vi "Restore Cursor Property.vi"(4 "Control Ref Cluster":T1, 6 "Update?":bool=TRUE, 8 "error in (no error)":errorcluster, 11 "2D Plot.lvclass in":refnum<class "2D Plot.lvclass">) -> (0 "error out":errorcluster, 3 "2D Plot.lvclass out":refnum<class "2D Plot.lvclass">)   [LabVIEW 2017, in "2D Plot.lvclass"]
uses:
  <vilib>/Math Plots/2D Math Plots/2D Plot/2D Plot/2D Plot.lvclass
  <vilib>/Math Plots/2D Math Plots/2D Plot/Action String/2DMathPlot Ctrl Act Cluster.ctl
  <vilib>/Math Plots/2D Math Plots/2D Plot/Action String/2DMathPlot State Class.ctl
  <vilib>/Math Plots/2D Math Plots/2D Plot/2D Plot/2D Plot.lvclass/2D Plot.ctl
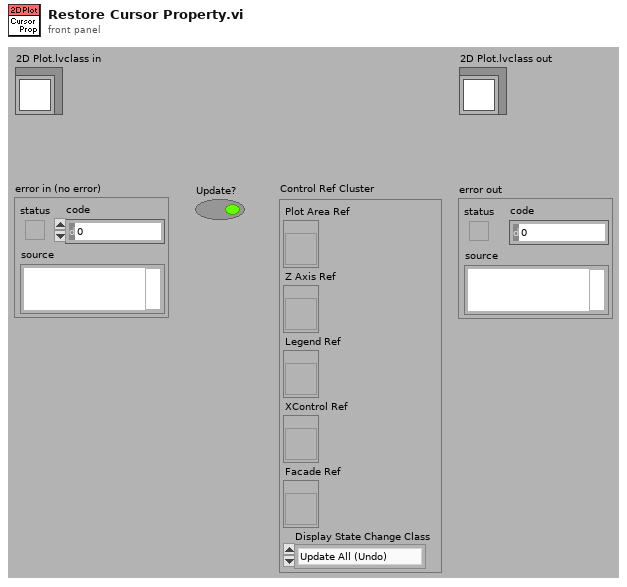
[diagram p1: front panel]
types:
  T1 = typedef "2DMathPlot Ctrl Act Cluster.ctl" = cluster{"Plot Area Ref":refnum<vi>, "Z Axis Ref":refnum<vi>, "Legend Ref":refnum<vi>, "XControl Ref":refnum<vi>, "Facade Ref":refnum<vi>, "Display State Change Class":T2}
  T2 = typedef "2DMathPlot State Class.ctl" = enum16{"Update All (Undo)", "Update General", "Update Appearance", "Update Format", "Update Scale", "Update Marker", "Update Cursor", "None"}
  T3 = typedef "LVCursorListTypeDef.ctl" = cluster{"Name":string, "Color":u32, "Style":u8, "Point Style":u8, "Name Visible":bool, "Allow Drag":bool, "Cursor Mode":u32, "Plot":i32, "Index":i32, "Position":cluster{"X":dbl, "Y":dbl}, "X Scale":u32, "Y Scale":u32, "Watch Plots":i32[], "Watch All Plots":bool, "Plot Area":i32, "Label Offset":cluster{"X":dbl, "Y":dbl}}[]
  T4 = cluster{"Cursor Selection Color":u32, "Line Style":u8, "Line Width":u8, "Visible":bool}[]
  T5 = cluster{"Name":string, "Color":u32, "Style":u8, "Point Style":u8, "Name Visible":bool, "Allow Drag":bool, "Cursor Mode":u32, "Plot":i32, "Index":i32, "Position":cluster{"X":dbl, "Y":dbl}, "X Scale":u32, "Y Scale":u32, "Watch Plots":i32[], "Watch All Plots":bool, "Plot Area":i32, "Label Offset":cluster{"X":dbl, "Y":dbl}}
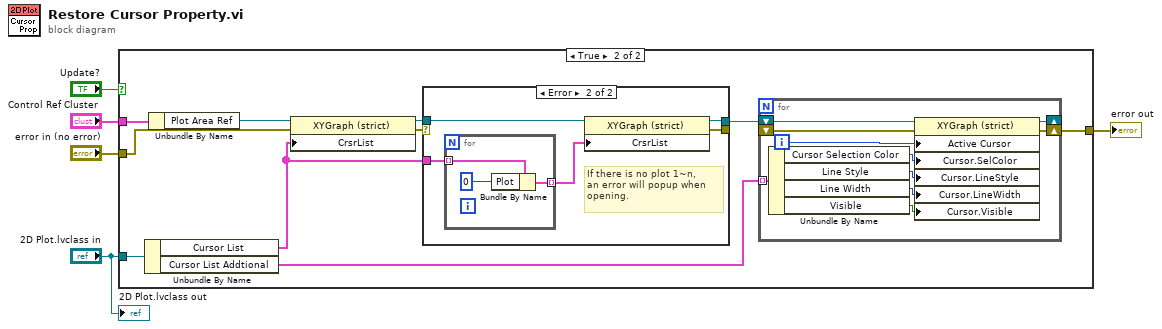
[diagram p0: block diagram]
diagram:
  n1 = case shown="True" "Update?" {
    tunnel: "Control Ref Cluster" -> [_ w14]
    tunnel: "error in (no error)" -> [w6 w12]
    tunnel: "2D Plot.lvclass in" -> [_ w11]
    tunnel: [w6 w7] -> w2
    frame False {
    }
    frame True {
      n2 = Unbundle By Name(w11) -> ("Cursor List"=w8:T3, "Cursor List Addtional"=w10:T4)
      n3 = Unbundle By Name(w14) -> ("Plot Area Ref"=w13:refnum<vi>)
      n4 = property class="XYGraph (strict)"(reference=w13, error in=w12, "CrsrList"=w8) -> (reference out=w16:refnum<vi>, error out=w15:errorcluster)
      n5 = case shown="Error" w15 {
        selector: w15 -> [w18 _]
        tunnel: [w18 w21] -> _
        tunnel: w16 -> [w17 w23]
        tunnel: [w17 w22] -> w9
        tunnel: w8 -> [_ w20]
        frame No Error {
        }
        frame Error {
          # "If there is no plot 1~n, \nan error will popup when \nopening."
          n6 = for {
            tunnel: w20 -> [w25] mode=indexing
            tunnel: [w24] -> w19 mode=indexing
            n7 = Bundle By Name(cluster=w25, "Plot"=0) -> (w24:T5)
          }
          n8 = property class="XYGraph (strict)"(reference=w23, "CrsrList"=w19) -> (reference out=w22:refnum<vi>, error out=w21:errorcluster)  [unwired: 1 in]
        }
      }
      n9 = for {
        tunnel: w10 -> [w35] mode=indexing
        shift-right: [w29] -> _
        shift-left: w9 -> [w30]
        shift-right: [w27] -> w7
        shift-left: _ -> [w28]
        i -> [w36]
        n10 = Unbundle By Name(w35) -> ("Cursor Selection Color"=w34:u32, "Line Style"=w33:u8, "Line Width"=w32:u8, "Visible"=w31:bool)
        n11 = property class="XYGraph (strict)"(reference=w30, error in=w28, "Active Cursor"=w36, "Cursor.SelColor"=w34, "Cursor.LineStyle"=w33, "Cursor.LineWidth"=w32, "Cursor.Visible"=w31) -> (reference out=w29:refnum<vi>, error out=w27:errorcluster)
      }
    }
  }
  "error out" <- w2
  "2D Plot.lvclass out" <- "2D Plot.lvclass in"
